vi "Operate.vi"(8 "error in (no error)":errorcluster, 11 "NumericOperation in":refnum<class "NumericOperation.lvclass">) -> (0 "error out":errorcluster, 2 "C":dbl, 3 "NumericOperation out":refnum<class "NumericOperation.lvclass">)   [LabVIEW 2021, in "Calculator.lvlib" / "NumericOperation.lvclass"]
doc: "This VI acts as a parent class method that is overrided between child classes."
uses:
  NumericOperation.lvclass
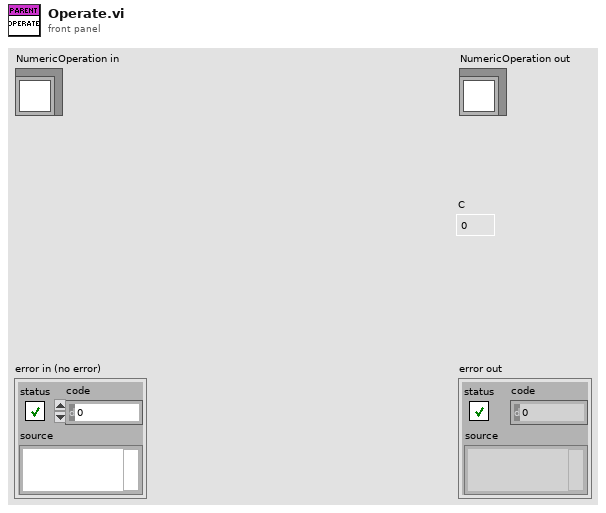
[diagram p1: front panel]
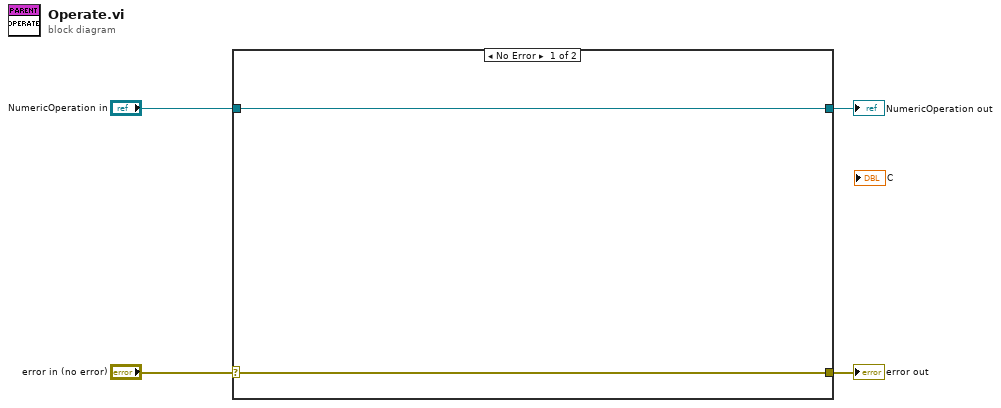
[diagram p0: block diagram]
diagram:
  n1 = case shown="No Error" "error in (no error)" {
    selector: "error in (no error)" -> [w5 w8]
    tunnel: [w5 w8] -> w3
    tunnel: [w6 w7] -> w1
    tunnel: "NumericOperation in" -> [w6 w7]
    frame No Error {
    }
    frame Error {
    }
  }
  "error out" <- w3
  "NumericOperation out" <- w1
